vi "Subscribe.vi"(4 "Excluded (None)":refnum<class>[](array[class]), 6 "Included (All)":refnum<class>[](array[class]), 8 "error in (no error)":errorcluster, 9 "Name":string, 10 "Receivers Enqueuer":refnum<class "Message Enqueuer.lvclass">, 11 "Pub Sub Message Channel in":refnum<class "Pub Sub Message Channel.lvclass">) -> (0 "error out":errorcluster, 2 "New Subscription":bool, 3 "Pub Sub Message Channel out":refnum<class "Pub Sub Message Channel.lvclass">)   [LabVIEW 2020, in "Actor Pub Sub Channels.lvlib" / "Pub Sub Message Channel.lvclass"]
uses:
  Pub Sub Message Channel.lvclass
  <vilib>/ActorFramework/Message Enqueuer/Message Enqueuer.lvclass
  Pub Sub Message Channel.lvclass/Pub Sub Message Channel.ctl
  <vilib>/ActorFramework/Message Queue/Message Queue.lvclass/Message Queue.ctl
  PubSub Status Reciever Interface Messages/Recieve New Subscription Msg/Receive New Subscription Msg.lvclass/Receive New Subscription Msg.ctl
  <vilib>/ActorFramework/Message Enqueuer/Message Enqueuer.lvclass/Message Enqueuer.ctl
  <vilib>/ActorFramework/Message Enqueuer/Enqueue.vi
  PubSub Status Reciever Interface Messages/Recieve New Subscription Msg/Receive New Subscription Msg.lvclass
  C:/Program Files (x86)/National Instruments/LabVIEW 2020/vi.lib/ActorFramework/Message/Message.lvclass
  <vilib>/ActorFramework/Message Priority Queue/Priority Enqueue.vi
  <vilib>/ActorFramework/Message Queue/Message Queue.lvclass
  <vilib>/ActorFramework/Message/Message.lvclass
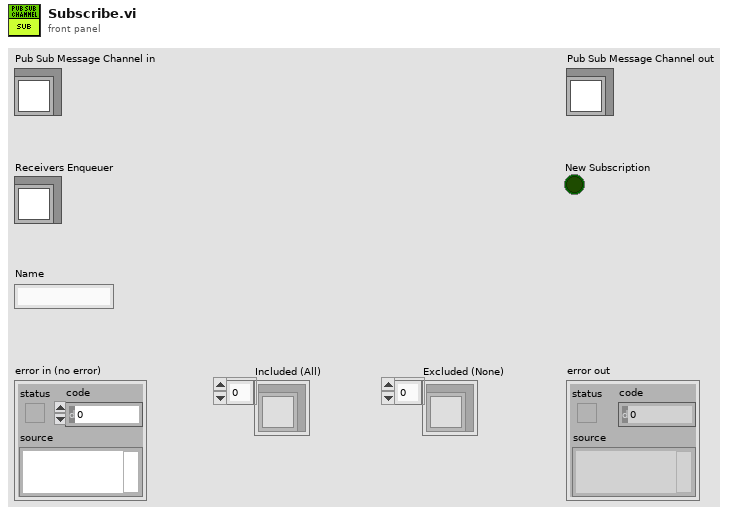
[diagram p1: front panel]
types:
  T1 = map{refnum<class "Message Enqueuer.lvclass">, cluster{"Name":string, "Included (All)":refnum<class "Message.lvclass">[], "Excluded (None)":refnum<class "Message.lvclass">[]}}
  T2 = cluster{"Name":string, "Included (All)":refnum<class>[], "Excluded (None)":refnum<class>[]}
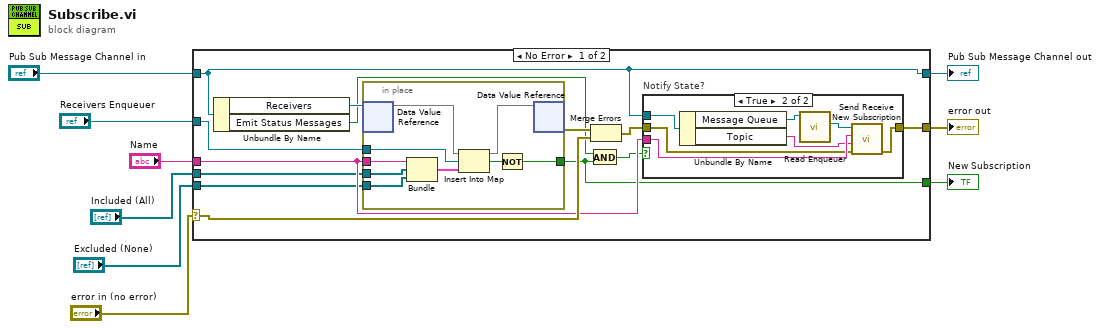
[diagram p0: block diagram]
diagram:
  n1 = case shown="No Error" "error in (no error)" {
    selector: "error in (no error)" -> [w22 w41]
    tunnel: [w13 w41] -> w8
    tunnel: [w18 w40] -> w6
    tunnel: "Pub Sub Message Channel in" -> [w18 w40]
    tunnel: "Receivers Enqueuer" -> [w20 _]
    tunnel: "Name" -> [w17 _]
    tunnel: [w12 _] -> w3
    tunnel: "Included (All)" -> [w11 _]
    tunnel: "Excluded (None)" -> [w10 _]
    frame No Error {
      n2 = Unbundle By Name(w18) -> ("Receivers"=w21:refnum<data-value>, "Emit Status Messages"=w15:bool)
      n3 = in-place {
        in-place-border: w20 -> [w37]
        in-place-border: w17 -> [w34]
        in-place-border: [w35] -> w12
        in-place-border: w11 -> [w33]
        in-place-border: w10 -> [w32]
        n4 = in-place-dvr #1(w21) -> (w39:T1)  [unwired: 1 out]
        n5 = Bundle("Name"=w34, "Included (All)"=w33, "Excluded (None)"=w32) -> (w31:T2)  [unwired: 1 in]
        n6 = Insert Into Map(map in=w39, key=w37, value=w31) -> (map out=w38:T1, key already included?=w36:bool)  [unwired: 1 out]
        n7 = Not(x=w36) -> (.not. x?=w35:bool)
        n8 = in-place-dvr #1(w38) -> (w19:errorcluster)  [unwired: 1 out]
      }
      n9 = And(x=w15, y=w12) -> (x .and. y?=w16:bool)
      n10 = Merge Errors(w19, w22) -> (w14:errorcluster)
      n11 = case "Notify State?" shown="True" w16 {
        tunnel: w18 -> [_ w30]
        tunnel: w17 -> [_ w27]
        tunnel: w14 -> [w23 w25]
        tunnel: [w23 w24] -> w13
        frame False {
        }
        frame True {
          n12 = Unbundle By Name(w30) -> ("Message Queue"=w29:refnum<class "Message Queue.lvclass">, "Topic"=w26:string)
          n13 = call <vilib>:"Read Enqueuer.vi"("Message Queue"=w29) -> ("Message Enqueuer"=w28:refnum<class "Message Enqueuer.lvclass">)  [unwired: 10 in]
          n14 = call "Send Receive New Subscription.vi"("error in (no error)"=w25, "Topic"=w26, "Name"=w27, "Message Enqueuer"=w28) -> ("error out"=w24:errorcluster)  [unwired: 6 in, 1 out]
        }
      }
    }
    frame Error {
    }
  }
  "error out" <- w8
  "Pub Sub Message Channel out" <- w6
  "New Subscription" <- w3
